vi "test_value change.vi"() -> ()   [LabVIEW 2019]
panel:
  out "Numeric":dbl
  in  "OK Button":bool
  in  "stop":bool
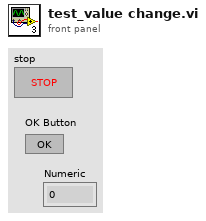
[diagram p1: front panel]
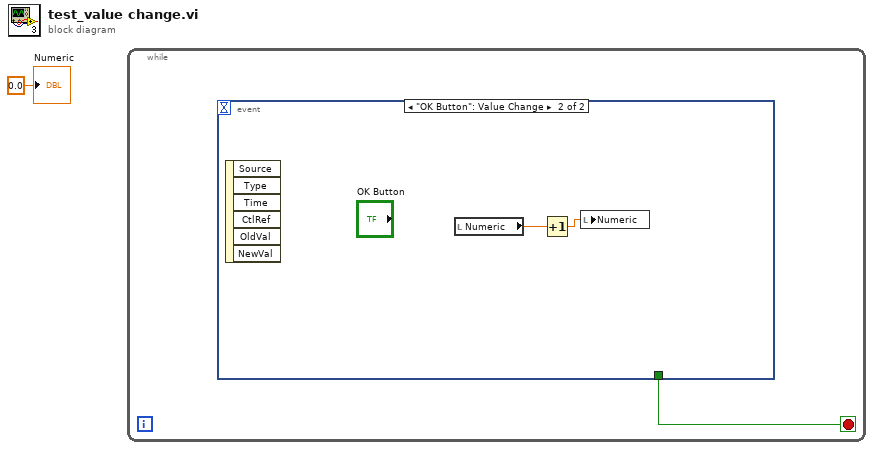
[diagram p0: block diagram]
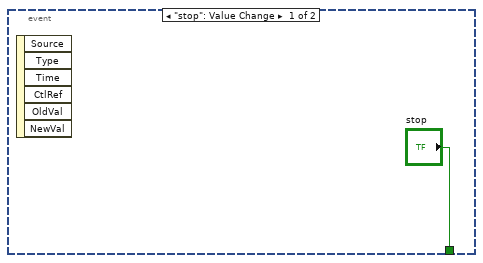
[diagram p2: hidden frame]
diagram:
  n1 = while {
    stop <- w2 stop-if-true
    n2 = event shown="[1] \"OK Button\": Value Change" {
      selector: _ -> [_ _]
      dyn-events: _ -> [_ _]
      timeout: _ -> [_ _]
      tunnel: ["stop" _] -> w2
      event "stop": Value Change {
        n3 = event-data() -> ()  [unwired: 1 in, 6 out]
      }
      event "OK Button": Value Change {
        n4 = event-data() -> ()  [unwired: 1 in, 6 out]
        n5 = local read "Numeric"() -> (w5:dbl)
        n6 = Increment(x=w5) -> (x+1=w4:dbl)
        n7 = local write "Numeric"(w4) -> ()
      }
    }
  }
  "Numeric" <- 0.0 ("Numeric")
